vi "JLMainUI.vi"(2 "JL_Buttons":T1, 8 "Error In":errorcluster, 9 "stop":bool, 11 "LED Update Rate (s)":dbl=0.25 caption="Delay Time (s)") -> (0 "Error Out":errorcluster, 10 "JL_Buttons.ctlJL_LEDs":T2)   [LabVIEW 2016]
uses:
  JL Dryer Tool Support/JL_LEDs/JL_LEDs.ctl
  <vilib>/Utility/error.llb/whitespace.ctl
  Automation/Product Specific/Clothes Care/Justice League/Product Testcode/Common/Type Defs/JL_Buttons.ctl
  Automation/Product Specific/Clothes Care/Justice League/Product Testcode/Common/Type Defs/JL_Encoder_ Position.ctl
panel:
  out "Label.Text":string
  in  "Soft Load box?":bool
  in  "Tab Control":T3(tab)
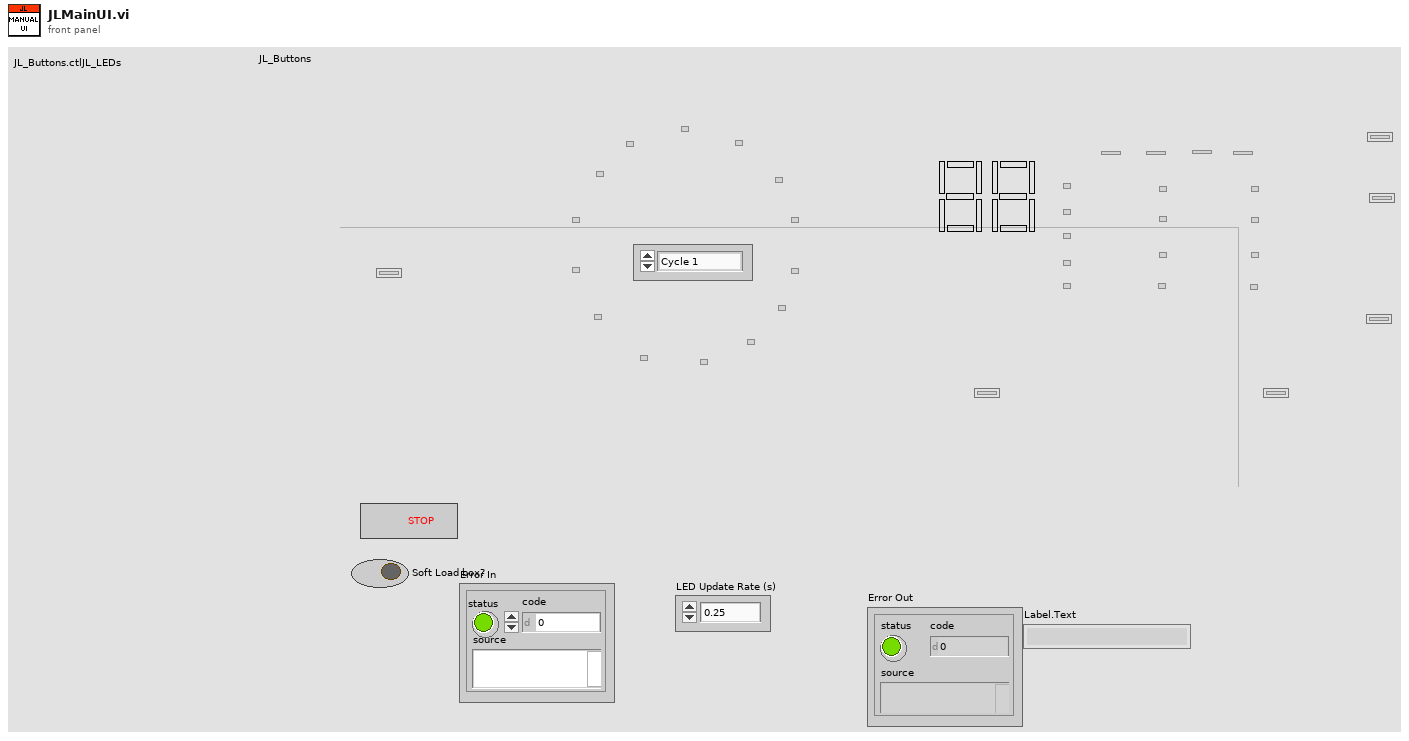
[diagram p1: front panel]
types:
  T1 = cluster{"SW204 -Damp Alert":bool, "SW203 - Volume":bool, "SW201 - My Cycle":bool, "SW202 - Delay Dry":bool, "SW209 - Time":bool, "SW207 - Level":bool, "SW205 - Temp":bool, "SW213 - Power":bool, "SW214 - Start/Pause":bool, "SW211 - eDry":bool, "SW210 - Add Time":bool, "SW208 - Sub Time":bool, "SW001 - Ex. Tumble":bool, "Cycle Selection 2":enum16{"Cycle 1", "Cycle 2", "Cycle 3", "Cycle 4", "Cycle 5", "Cycle6", "Cycle 7", "Cycle 8", "Cycle 9", "Cycle 10", "Cycle 11", "Cycle 12", "Cycle 13"}}
  T2 = typedef "JL_LEDs.ctl" = cluster{"Z102 - Start":bool, "Z301 - Encoder 0":bool, "Z302- Encoder 13":bool, "Z303 - Encoder 12":bool, "Z304 - Encoder 11":bool, "Z305 - Encoder 10":bool, "Z306 - Encoder 09":bool, "Z307 - Encoder 08":bool, "Z308- Encoder 07":bool, "Z309 - Encoder 06":bool, "Z310 - Encoder 05":bool, "Z311 - Encoder 04":bool, "Z312 - Encoder 03":bool, "Z313 - Encoder 02":bool, "Z314 - Encoder 01":bool, "Z136 - Pause":bool, "Z137 - Pause":bool, "Z138 - Lock Controls":bool, "Z139 - Lock Controls":bool, "Z140 - Lock Controls":bool, "Z326 - Sensing 1":bool, "Z331 -Sensing 2":bool, "Z353 - Sensing 3":bool, "Delay":bool, "Drying":bool, "Cooling":bool, "Done":bool, "Z101 - Hot":bool, "Z368 - Default Time 4":bool, "Z369 - Default Time 3":bool, "Z372 -Default Time 2":bool, "Z373 - Default Time 1":bool, "Z375 - Default Time 0":bool, "Z383 - More Dry":bool, "Z370 - Dry":bool, "Z388 - Less Dry":bool, "Z391 - Damp":bool, "Z384 - High":bool, "Z385 - Medium":bool, "Z388 - Extra Low":bool, "Z376 - No Heat":bool, "Z351 - Damp Alert":bool, "Z361 - Extended Tumble":bool, "Z358 - eDry":bool, "Z348 -My Cycle":bool, "Z349 - Delay Dry":bool, "Z327 - Clean Lint Filter 1":bool, "Z330 - Clean Lint Filter 2":bool, "Z342 - Clean Lint Filter 3":bool, "Z179 - Pause":bool, "Z109":bool, "Z110":bool, "Z123":bool, "Z124":bool, "Z140":bool, "Unused0":bool, "Unused1":bool, "Unused2":bool, "Unused3":bool, "Channel_Off":bool, "Channel_Cycle_Unmapped":bool, "Z319 - SSD1:G":bool, "Z317 - SSD1:A":bool, "Z318 - SSD1:B":bool, "Z323 - SSD1:F":bool, "Z321 - SSD1:D":bool, "Z320 - SSD1:C":bool, "Z322 - SSD1:E":bool, "Z335 - SSD2:G":bool, "Z333 - SSD2:A":bool, "Z334 - SSD2:B":bool, "Z338 - SSD2:F":bool, "Z336 - SSD2:D":bool, "Z345 - SSD2:C":bool, "Z337 - SSD2:E":bool}
  T3 = enum32{"Normal", "Pause ", "Lock", "Sensing", "Lint Filter"}
  T4 = typedef "JL_Buttons.ctl" = enum16{"Power", "Start / Pause ", "Temp Option ", "Dryness Level", "Time Option", "Time Increment ", "Time Decrement ", "MyCycle", "eDry ", "Delay", "Extended Tumble", "Control Lock", "Volume/Signal", "Damp Alert / Drum Light", "Unused", "(SW213)", "(SW322)", "Clear / Reset"}
  T5 = typedef "JL_Encoder_ Position.ctl" = enum16{"Position 0", "Position 1", "Position 2", "Position 3", "Position 4", "Position 5", "Position 6", "Position 7", "Position 8", "Position 9", "Position 10", "Position 11", "Position 12", "Position 13", "Position 14", "Clear / Reset"}
  T6 = typedef "whitespace.ctl" = u16
  T7 = enum16{"Cycle 1", "Cycle 2", "Cycle 3", "Cycle 4", "Cycle 5", "Cycle6", "Cycle 7", "Cycle 8", "Cycle 9", "Cycle 10", "Cycle 11", "Cycle 12", "Cycle 13"}
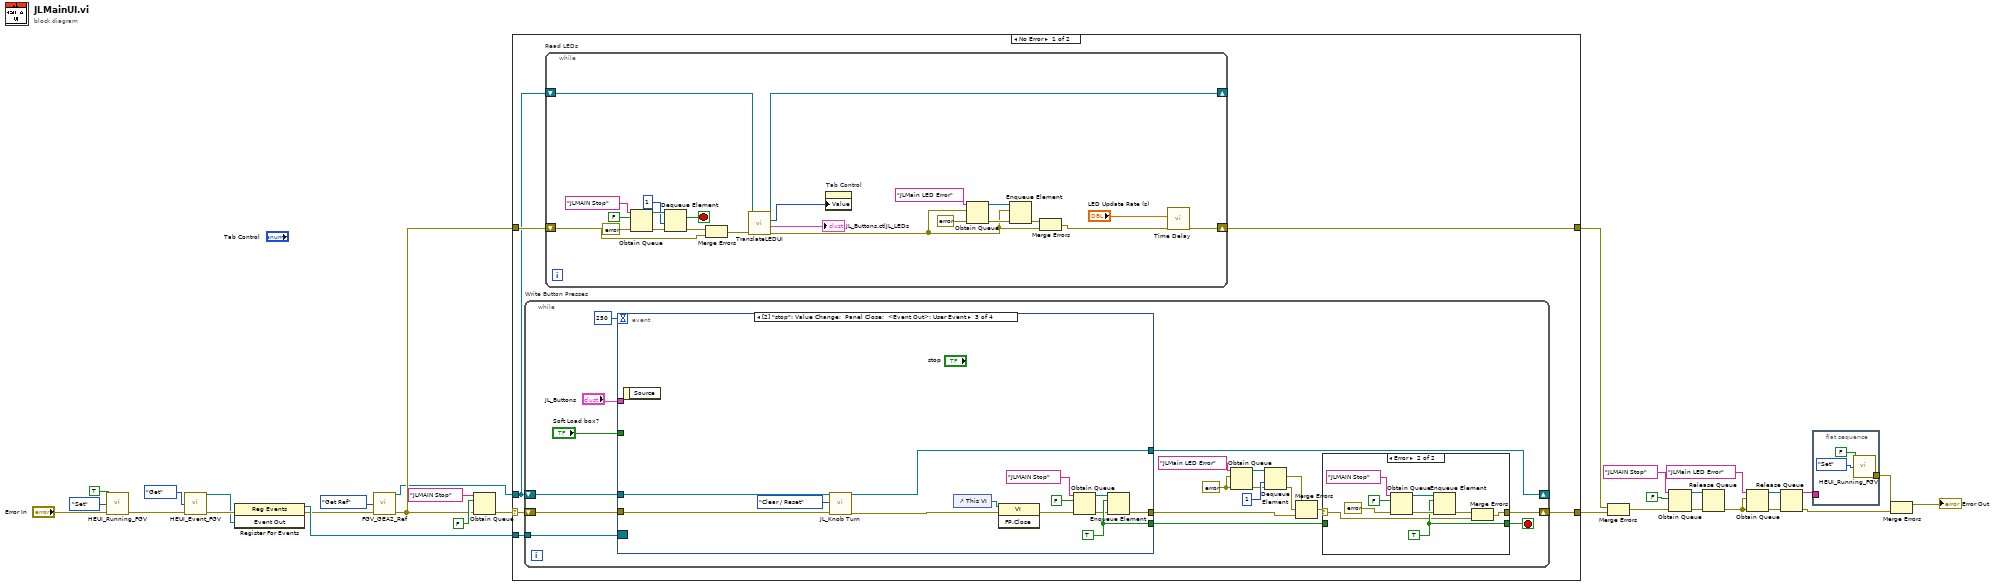
[diagram p0: block diagram]
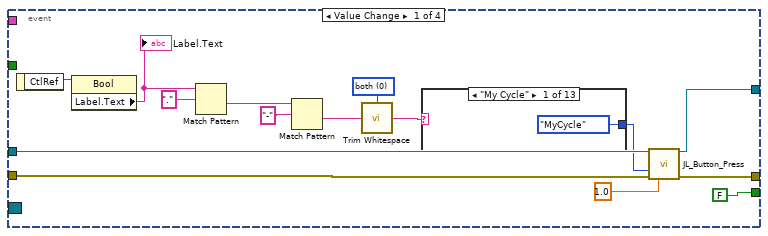
[diagram p3: hidden frame]
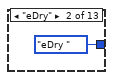
[diagram p4: hidden frame]
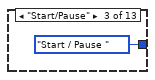
[diagram p5: hidden frame]
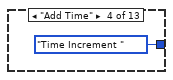
[diagram p6: hidden frame]
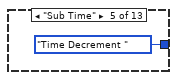
[diagram p7: hidden frame]
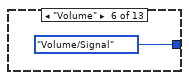
[diagram p8: hidden frame]
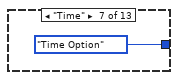
[diagram p9: hidden frame]
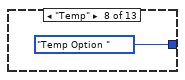
[diagram p10: hidden frame]
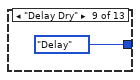
[diagram p11: hidden frame]
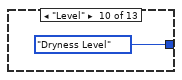
[diagram p12: hidden frame]
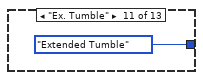
[diagram p13: hidden frame]
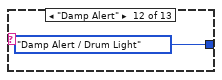
[diagram p14: hidden frame]
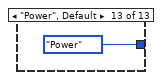
[diagram p15: hidden frame]
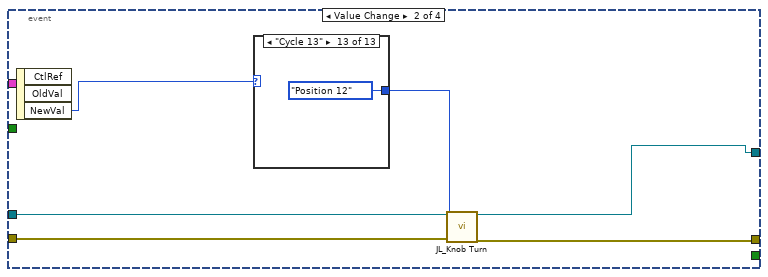
[diagram p16: hidden frame]
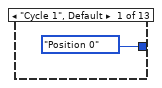
[diagram p17: hidden frame]
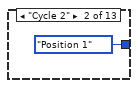
[diagram p18: hidden frame]
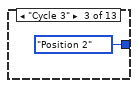
[diagram p19: hidden frame]
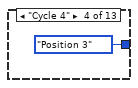
[diagram p20: hidden frame]
diagram:
  n1 = call "HEUI_Running_FGV.vi"("Running?"=TRUE, "Action"=enum16{"Get", "Set"}."Set", "Error In"="Error In") -> ("Error Out"=w5:errorcluster)  [unwired: 11 in, 1 out]
  n2 = call "HEUI_Event_FGV.vi"("Action"=enum16{"Get", "Set"}."Get", "Error In"=w5) -> ("Event Out"=w15:refnum<user-event>, "Error Out"=w16:errorcluster)  [unwired: 12 in]
  n3 = register-events(error in=w16, w15) -> (reference out=w18:refnum<event-registration>, error out=w11:errorcluster)  [unwired: 1 in]
  n4 = call "FGV_GEA2_Ref.vi"("Action"=enum16{"Set Ref", "Get Ref"}."Get Ref", "Error In"=w11) -> ("GEA2 Reference Out"=w9:refnum<k24>, "Error Out"=w10:errorcluster)  [unwired: 12 in]
  n5 = Obtain Queue(name (unnamed)="JLMAIN Stop", element data type=FALSE ("stop"), error in (no error)=w10) -> (error out=w23:errorcluster)  [unwired: 2 in, 2 out]
  n6 = case shown="No Error" w23 {
    selector: w23 -> [w32 w154]
    tunnel: w9 -> [w33 _]
    tunnel: [w36 errorcluster {"status"=FALSE, "code"=0, "source"=""} ("error out")] -> w30
    tunnel: [w35 w154] -> w13
    tunnel: w10 -> [w34 _]
    tunnel: w18 -> [w31 _]
    frame No Error {
      n7 = while "Write Button Presses" {
        shift-right: [w75] -> w35
        shift-left: w32 -> [w78]
        shift-right: [w76] -> _
        shift-left: w33 -> [w77]
        tunnel: w31 -> [w62]
        stop <- w73 stop-if-true
        w67 = errorcluster {"status"=FALSE, "code"=0, "source"=""} ("error in (no error)")
        n8 = event shown="[2] \"stop\": Value Change;  Panel Close;  <Event Out>: User Event" {
          selector: w62 -> [_ _ _ _]
          dyn-events: _ -> [_ _ _ _]
          timeout: 250 -> [_ _ _ _]
          tunnel: [w100 w121 w148 w151] -> w65
          tunnel: w78 -> [w102 w120 w139 w151]
          tunnel: w77 -> [w103 w123 w138 w152]
          tunnel: [w101 w122 w141 w152] -> w76
          tunnel: [FALSE ("stop") _ w147 FALSE ("stop")] -> w74
          tunnel: "JL_Buttons" -> [_ _ _ _]
          tunnel: "Soft Load box?" -> [_ _ _ _]
          event "JL_Buttons.SW001 - Ex. Tumble", "JL_Buttons.SW209 - Time", "JL_Buttons.SW205 - Temp", "JL_Buttons.SW202 - Delay Dry", "JL_Buttons.SW207 - Level", "JL_Buttons.SW214 - Start/Pause", "JL_Buttons.SW211 - eDry", "JL_Buttons.SW210 - Add Time", "JL_Buttons.SW208 - Sub Time", "JL_Buttons.SW204 -Damp Alert", "JL_Buttons.SW203 - Volume", "JL_Buttons.SW213 - Power", "JL_Buttons.SW201 - My Cycle": Value Change {
            w96 = T6 0 items=["both", "start of string", "end of string"] ("location (both)")
            n9 = event-data() -> ("CtlRef"=w92:refnum<vi>)  [unwired: 1 in]
            n10 = property class="Bool"(reference=w92) -> ("Label.Text"=w98:string)  [unwired: 1 in, 2 out]
            "Label.Text" <- w98
            n11 = Match Pattern(string=w98, regular expression=".") -> (after substring=w95:string)  [unwired: 1 in, 3 out]
            n12 = Match Pattern(string=w95, regular expression="-") -> (after substring=w94:string)  [unwired: 1 in, 3 out]
            n13 = call <vilib>:"Trim Whitespace.vi"("string"=w94, "location (both)"=w96) -> ("trimmed string"=w93:string)
            n14 = case shown="\"My Cycle\"" w93 {
              tunnel: [JL_Buttons."MyCycle" ("Button") JL_Buttons."eDry " ("Button") JL_Buttons."Start / Pause " ("Button") JL_Buttons."Time Increment " ("Button") JL_Buttons."Time Decrement " ("Button") JL_Buttons."Volume/Signal" ("Button") JL_Buttons."Time Option" ("Button") JL_Buttons."Temp Option " ("Button") JL_Buttons."Delay" ("Button") JL_Buttons."Dryness Level" ("Button") JL_Buttons."Extended Tumble" ("Button") JL_Buttons."Damp Alert / Drum Light" ("Button") JL_Buttons."Power" ("Button")] -> w90
              frame "My Cycle" {
              }
              frame "eDry" {
              }
              frame "Start/Pause" {
              }
              frame "Add Time" {
              }
              frame "Sub Time" {
              }
              frame "Volume" {
              }
              frame "Time" {
              }
              frame "Temp" {
              }
              frame "Delay Dry" {
              }
              frame "Level" {
              }
              frame "Ex. Tumble" {
              }
              frame "Damp Alert" {
              }
              frame "Power", Default {
              }
            }
            n15 = call "JL_Button_Press.vi"("GEA2 Reference In"=w103, "Button"=w90, "Error In"=w102, "Hold Time (s)"=1.0) -> ("GEA2 Reference Out"=w101:refnum<k24>, "Error Out"=w100:errorcluster)  [unwired: 10 in]
          }
          event "JL_Buttons.Cycle Selection 2": Value Change {
            n16 = event-data() -> ("NewVal"=w119:T7)  [unwired: 1 in, 2 out]
            n17 = case shown="\"Cycle 13\"" w119 {
              tunnel: [JL_Encoder__Position."Position 0" ("Knob Position") JL_Encoder__Position."Position 1" ("Knob Position") JL_Encoder__Position."Position 2" ("Knob Position") JL_Encoder__Position."Position 3" ("Knob Position") JL_Encoder__Position."Position 4" ("Knob Position") JL_Encoder__Position."Position 5" ("Knob Position") JL_Encoder__Position."Position 6" ("Knob Position") JL_Encoder__Position."Position 7" ("Knob Position") JL_Encoder__Position."Position 8" ("Knob Position") JL_Encoder__Position."Position 9" ("Knob Position") JL_Encoder__Position."Position 10" ("Knob Position") JL_Encoder__Position."Position 11" ("Knob Position") JL_Encoder__Position."Position 12" ("Knob Position")] -> w118
              frame "Cycle 1", Default {
              }
              frame "Cycle 2" {
              }
              frame "Cycle 3" {
              }
              frame "Cycle 4" {
              }
              frame "Cycle 5" {
              }
              frame "Cycle6" {
              }
              frame "Cycle 7" {
              }
              frame "Cycle 8" {
              }
              frame "Cycle 9" {
              }
              frame "Cycle 10" {
              }
              frame "Cycle 11" {
              }
              frame "Cycle 12" {
              }
              frame "Cycle 13" {
              }
            }
            n18 = call "JL_Knob Turn.vi"("GEA2 Reference In"=w123, "Knob Position"=w118, "Error In"=w120) -> ("GEA2 Reference Out"=w122:refnum<k24>, "Error Out"=w121:errorcluster)  [unwired: 15 in]
          }
          event "stop": Value Change; Panel Close; User Event {
            w147 = TRUE ("stop")
            n19 = event-data() -> ()  [unwired: 1 in, 1 out]
            n20 = call "JL_Knob Turn.vi"("GEA2 Reference In"=w138, "Knob Position"=JL_Encoder__Position."Clear / Reset", "Error In"=w139) -> ("GEA2 Reference Out"=w141:refnum<k24>, "Error Out"=w140:errorcluster)  [unwired: 15 in]
            n21 = control-ref of="This VI"() -> (w149:refnum<vi>)
            n22 = invoke class="VI" method="FP.Close"(reference=w149, error in=w140) -> (error out=w146:errorcluster)  [unwired: 1 in, 2 out]
            n23 = Obtain Queue(name (unnamed)="JLMAIN Stop", element data type=FALSE ("stop"), error in (no error)=w146) -> (queue out=w144:refnum<queue>, error out=w145:errorcluster)  [unwired: 2 in, 1 out]
            n24 = Enqueue Element(queue=w144, element=w147, error in (no error)=w145) -> (error out=w148:errorcluster)  [unwired: 1 in, 2 out]
          }
          event Timeout {
            n25 = event-data() -> ()  [unwired: 1 in, 3 out]
          }
        }
        n26 = Obtain Queue(name (unnamed)="JLMain LED Error", element data type=w67, error in (no error)=w67) -> (queue out=w69:refnum<queue>, error out=w70:errorcluster)  [unwired: 2 in, 1 out]
        n27 = Dequeue Element(queue=w69, timeout in ms (-1)=1, error in (no error)=w70) -> (element=w63:errorcluster, error out=w64:errorcluster)  [unwired: 2 out]
        n28 = Merge Errors(w63, w64, w65) -> (w68:errorcluster)
        n29 = case shown="Error" w68 {
          selector: w68 -> [w80 w82]
          tunnel: [w80 w84] -> w75
          tunnel: w74 -> [w79 _]
          tunnel: [w79 w85] -> w73
          frame No Error {
          }
          frame Error {
            w85 = TRUE ("stop")
            n30 = Obtain Queue(name (unnamed)="JLMAIN Stop", element data type=FALSE ("stop"), error in (no error)=errorcluster {"status"=FALSE, "code"=0, "source"=""}) -> (queue out=w88:refnum<queue>, error out=w89:errorcluster)  [unwired: 2 in, 1 out]
            n31 = Enqueue Element(queue=w88, element=w85, error in (no error)=w89) -> (error out=w83:errorcluster)  [unwired: 1 in, 2 out]
            n32 = Merge Errors(w83, w82) -> (w84:errorcluster)
          }
        }
      }
      n33 = while "Read LEDs" {
        shift-right: [w59] -> w36
        shift-left: w34 -> [w43]
        shift-right: [w37] -> _
        shift-left: w33 -> [w40]
        stop <- w57 stop-if-true
        n34 = Obtain Queue(name (unnamed)="JLMAIN Stop", element data type=FALSE ("stop"), error in (no error)=errorcluster {"status"=FALSE, "code"=0, "source"=""}) -> (queue out=w56:refnum<queue>, error out=w55:errorcluster)  [unwired: 2 in, 1 out]
        n35 = Dequeue Element(queue=w56, timeout in ms (-1)=1, error in (no error)=w55) -> (element=w57:bool, error out=w45:errorcluster)  [unwired: 2 out]
        n36 = Merge Errors(w45, w43) -> (w39:errorcluster)
        n37 = call "TranslateLEDUI.vi"("error in (no error)"=w39, "GEA2 Reference In"=w40) -> ("error out"=w38:errorcluster, "JL_Buttons.ctlJL_LEDs 2"=→"JL_Buttons.ctlJL_LEDs":T2, "Tab Control"=w42:T3, "GEA2 Reference Out"=w37:refnum<k24>)  [unwired: 4 in, 2 out]
        n38 = property on="Tab Control" class="TabCtl (strict)"("Value"=w42) -> ()  [unwired: 2 in, 2 out]
        n39 = Obtain Queue(name (unnamed)="JLMain LED Error", element data type=w38, error in (no error)=errorcluster {"status"=FALSE, "code"=0, "source"=""}) -> (queue out=w50:refnum<queue>, error out=w49:errorcluster)  [unwired: 2 in, 1 out]
        n40 = Enqueue Element(queue=w50, element=w38, error in (no error)=w49) -> (error out=w48:errorcluster)  [unwired: 1 in, 2 out]
        n41 = Merge Errors(w48, w38) -> (w47:errorcluster)
        n42 = call "Time Delay"("error in (no error)"=w47, "Delay Time (s)"="LED Update Rate (s)") -> ("error out"=w59:errorcluster)  [unwired: 9 in]
      }
    }
    frame Error {
    }
  }
  n43 = Merge Errors(w30, w13) -> (w14:errorcluster)
  n44 = Obtain Queue(name (unnamed)="JLMAIN Stop", element data type=FALSE ("stop"), error in (no error)=w14) -> (queue out=w24:refnum<queue>, error out=w25:errorcluster)  [unwired: 2 in, 1 out]
  n45 = Release Queue(queue=w24, error in (no error)=w25) -> (error out=w19:errorcluster)  [unwired: 1 in, 2 out]
  n46 = Obtain Queue(name (unnamed)="JLMain LED Error", element data type=w19, error in (no error)=w19) -> (queue out=w22:refnum<queue>, error out=w21:errorcluster)  [unwired: 2 in, 1 out]
  n47 = Release Queue(queue=w22, error in (no error)=w21) -> (queue name=w1:string, error out=w4:errorcluster)  [unwired: 1 in, 1 out]
  n48 = flat-sequence {
    tunnel: [w155] -> w3
    tunnel: w1 -> [_]
    frame #0 {
      n49 = call "HEUI_Running_FGV.vi"("Running?"=FALSE, "Action"=enum16{"Get", "Set"}."Set") -> ("Error Out"=w155:errorcluster)  [unwired: 12 in, 1 out]
    }
  }
  n50 = Merge Errors(w3, w4) -> (→"Error Out":errorcluster)
